vi "Config FGV.vi"(8 "Error In":errorcluster, 10 "Application Configuration Input Helper":T1, 11 "Action":T3) -> (0 "Error Out":errorcluster, 2 "Full Application Configuration":T1, 3 "Current Project Configuration":T2)   [LabVIEW 2014, in "i3-docs.lvlib"]
uses:
  i3-docs.lvlib
  Controls/config_fgv_actions.ctl
  Controls/config.ctl
  Controls/current_config.ctl
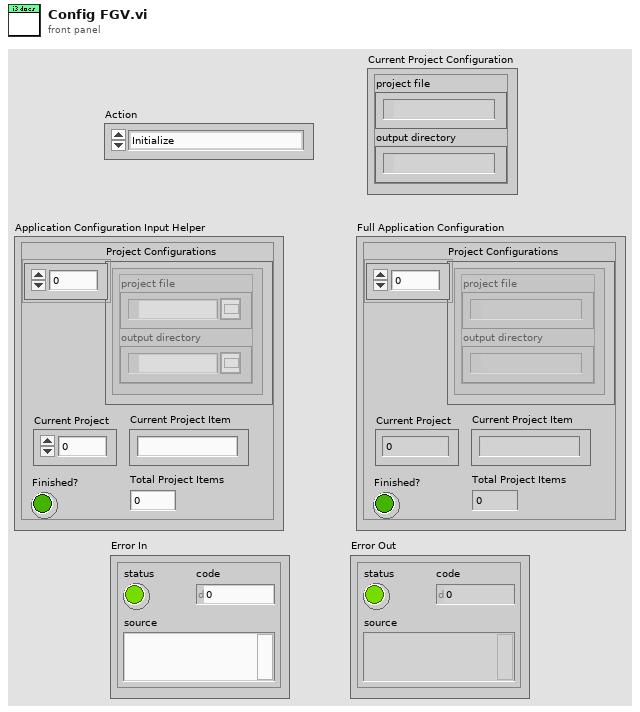
[diagram p1: front panel]
types:
  T1 = typedef "i3-docs.lvlib/config.ctl" = cluster{"Current Project":i32, "Project Configurations":T2[], "Current Project Item":string, "Finished?":bool, "Total Project Items":i32}
  T2 = typedef "i3-docs.lvlib/current_config.ctl" = cluster{"project file":path, "output directory":path}
  T3 = typedef "i3-docs.lvlib/config_fgv_actions.ctl" = enum16{"Initialize", "Set Current Project", "Get Current Config", "Set Current Project Item", "Finished"}
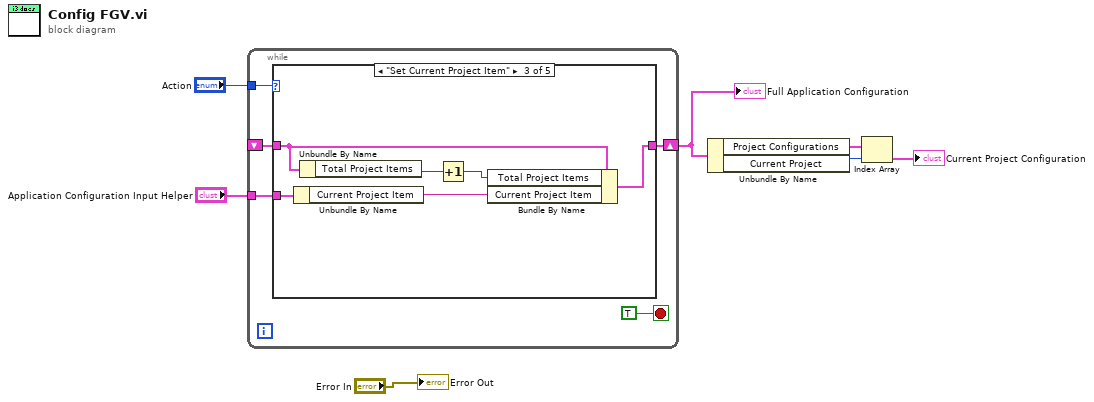
[diagram p0: block diagram]
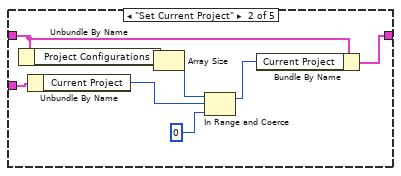
[diagram p3: hidden frame]
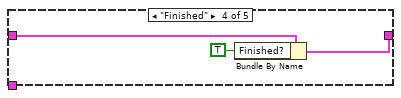
[diagram p4: hidden frame]
diagram:
  n1 = while {
    tunnel: "Action" -> [w11]
    shift-right: [w10] -> w6
    shift-left: _ -> [w9]
    tunnel: "Application Configuration Input Helper" -> [w8]
    stop <- TRUE stop-if-true
    n2 = case shown="\"Set Current Project Item\"" w11 {
      tunnel: [w13 w21 w27 w30 w31] -> w10
      tunnel: w9 -> [_ w20 w24 w29 w31]
      tunnel: w8 -> [w13 w15 w26 _ _]
      frame "Initialize" {
      }
      frame "Set Current Project" {
        n3 = Unbundle By Name(w20) -> ("Project Configurations"=w18:T2[])
        n4 = Unbundle By Name(w15) -> ("Current Project"=w14:i32)
        n5 = Array Size(array=w18) -> (size(s)=w19:i32)
        n6 = In Range and Coerce(upper limit=w19, x=w14, lower limit=0) -> (coerced(x)=w16:i32)  [unwired: 1 out]
        n7 = Bundle By Name(cluster=w20, "Current Project"=w16) -> (w21:T1)
      }
      frame "Set Current Project Item" {
        n8 = Unbundle By Name(w26) -> ("Current Project Item"=w25:string)
        n9 = Unbundle By Name(w24) -> ("Total Project Items"=w23:i32)
        n10 = Increment(x=w23) -> (x+1=w22:i32)
        n11 = Bundle By Name(cluster=w24, "Total Project Items"=w22, "Current Project Item"=w25) -> (w27:T1)
      }
      frame "Finished" {
        n12 = Bundle By Name(cluster=w29, "Finished?"=TRUE) -> (w30:T1)
      }
      frame "Get Current Config" {
      }
    }
  }
  "Full Application Configuration" <- w6
  n13 = Unbundle By Name(w6) -> ("Project Configurations"=w5:T2[], "Current Project"=w4:i32)
  n14 = Index Array(array=w5, index=w4) -> (element=→"Current Project Configuration":T2)
  "Error Out" <- "Error In"
